vi "experiment control.vi"() -> ()   [LabVIEW 2012] (continued)
                          n671 = Enqueue Element At Opposite End(queue=w1523, element=w1521) -> ()  [unwired: 2 in, 3 out]
                        }
                        frame "Lasers" {
                          n672 = call "seek_tag.vi"("error in"=w1562, "Name"=w1563, "refnum"=w1561) -> ("error out"=w1559:errorcluster, "error"=w1552:string, "refnum"=w1560:refnum<file>)  [unwired: 6 in]
                          n673 = local read "Toptica"() -> (w1547:T19)
                          n674 = local read "Jessica"() -> (w1551:T17)
                          n675 = local read "Bertha"() -> (w1550:T22)
                          n676 = local read "Stella"() -> (w1548:T20)
                          n677 = local read "Cora"() -> (w1549:T21)
                          n678 = Concatenate Strings("Debug: Console >> " ("prompt (Open existing file)"), w1552) -> (w1543:string)
                          n679 = Bundle("Jessica"=w1551, "Bertha"=w1550, "Cora"=w1549, "Stella"=w1548, "Toptica"=w1547) -> (w1546:T88)  [unwired: 1 in]
                          n680 = call "ubinary.vi"("Cluster"=w1546) -> ("Header"=w1564:cluster{"Element Names":string[], u8[]})  [unwired: 9 in, 1 out]
                          n681 = Bundle("Header"=w1564, w1546) -> (w1557:T89)  [unwired: 1 in]
                          n682 = Read from Binary File(5:w1557, 8:w1559, 9:T45."native, host order" ("byte order (0:big-endian, network order)"), 11:w1560) -> (0:w1554:errorcluster, 2:w1555:T89, 3:w1556:refnum<file>)  [unwired: 2 in, 1 out]
                          n683 = case shown="No Error" w1554 {
                            tunnel: w1555 -> [w1571 _]
                            frame No Error {
                              n684 = Unbundle(w1571) -> (w1570:T88)  [unwired: 1 out]
                              n685 = Unbundle By Name(w1570) -> ("Jessica"=w1569:T17, "Bertha"=w1568:T22, "Cora"=w1567:T21, "Stella"=w1566:T20, "Toptica"=w1565:T19)
                              n686 = local write "Toptica"(w1565) -> ()
                              n687 = local write "Bertha"(w1568) -> ()
                              n688 = local write "Cora"(w1567) -> ()
                              n689 = local write "Stella"(w1566) -> ()
                              n690 = local write "Jessica"(w1569) -> ()
                            }
                            frame Error {
                            }
                          }
                          n691 = Enqueue Element At Opposite End(queue=w1544, element=w1543) -> ()  [unwired: 2 in, 3 out]
                        }
                        frame "AOM DDS" {
                          n692 = call "seek_tag.vi"("error in"=w1587, "Name"=w1588, "refnum"=w1586) -> ("error out"=w1584:errorcluster, "error"=w1577:string, "refnum"=w1585:refnum<file>)  [unwired: 6 in]
                          n693 = local read "DDS"() -> (w1576:T25)
                          n694 = Concatenate Strings("Debug: Console >> " ("prompt (Open existing file)"), w1577) -> (w1573:string)
                          n695 = Bundle("DDS"=w1576) -> (w1575:T66)  [unwired: 1 in]
                          n696 = call "ubinary.vi"("Cluster"=w1575) -> ("Header"=w1589:cluster{"Element Names":string[], u8[]})  [unwired: 9 in, 1 out]
                          n697 = Bundle("Header"=w1589, w1575) -> (w1582:T67)  [unwired: 1 in]
                          n698 = Read from Binary File(5:w1582, 8:w1584, 9:T45."native, host order" ("byte order (0:big-endian, network order)"), 11:w1585) -> (0:w1579:errorcluster, 2:w1580:T67, 3:w1581:refnum<file>)  [unwired: 2 in, 1 out]
                          n699 = case shown="No Error" w1579 {
                            tunnel: w1580 -> [w1592 _]
                            frame No Error {
                              n700 = Unbundle(w1592) -> (w1591:T66)  [unwired: 1 out]
                              n701 = Unbundle By Name(w1591) -> ("DDS"=w1590:T25)
                              n702 = local write "DDS"(w1590) -> ()
                            }
                            frame Error {
                            }
                          }
                          n703 = Enqueue Element At Opposite End(queue=w1572, element=w1573) -> ()  [unwired: 2 in, 3 out]
                        }
                        frame "Trap DDS" {
                          n704 = call "seek_tag.vi"("error in"=w1608, "Name"=w1609, "refnum"=w1607) -> ("error out"=w1605:errorcluster, "error"=w1598:string, "refnum"=w1606:refnum<file>)  [unwired: 6 in]
                          n705 = local read "Trap DDS"() -> (w1597:T26)
                          n706 = Concatenate Strings("Debug: Console >> " ("prompt (Open existing file)"), w1598) -> (w1594:string)
                          n707 = Bundle("Trap DDS"=w1597) -> (w1596:T68)  [unwired: 1 in]
                          n708 = call "ubinary.vi"("Cluster"=w1596) -> ("Header"=w1610:cluster{"Element Names":string[], u8[]})  [unwired: 9 in, 1 out]
                          n709 = Bundle("Header"=w1610, w1596) -> (w1603:T69)  [unwired: 1 in]
                          n710 = Read from Binary File(5:w1603, 8:w1605, 9:T45."native, host order" ("byte order (0:big-endian, network order)"), 11:w1606) -> (0:w1600:errorcluster, 2:w1601:T69, 3:w1602:refnum<file>)  [unwired: 2 in, 1 out]
                          n711 = case shown="No Error" w1600 {
                            tunnel: w1601 -> [w1613 _]
                            frame No Error {
                              n712 = Unbundle(w1613) -> (w1612:T68)  [unwired: 1 out]
                              n713 = Unbundle By Name(w1612) -> ("Trap DDS"=w1611:T26)
                              n714 = local write "Trap DDS"(w1611) -> ()
                            }
                            frame Error {
                            }
                          }
                          n715 = Enqueue Element At Opposite End(queue=w1593, element=w1594) -> ()  [unwired: 2 in, 3 out]
                        }
                        frame "Wavemaster" {
                          n716 = call "seek_tag.vi"("error in"=w1629, "Name"=w1630, "refnum"=w1628) -> ("error out"=w1626:errorcluster, "error"=w1619:string, "refnum"=w1627:refnum<file>)  [unwired: 6 in]
                          n717 = local read "Wavemaster"() -> (w1618:T23)
                          n718 = Concatenate Strings("Debug: Console >> " ("prompt (Open existing file)"), w1619) -> (w1614:string)
                          n719 = Bundle("Wavemaster"=w1618) -> (w1617:T76)  [unwired: 1 in]
                          n720 = call "ubinary.vi"("Cluster"=w1617) -> ("Header"=w1631:cluster{"Element Names":string[], u8[]})  [unwired: 9 in, 1 out]
                          n721 = Bundle("Header"=w1631, w1617) -> (w1624:T77)  [unwired: 1 in]
                          n722 = Read from Binary File(5:w1624, 8:w1626, 9:T45."native, host order" ("byte order (0:big-endian, network order)"), 11:w1627) -> (0:w1621:errorcluster, 2:w1622:T77, 3:w1623:refnum<file>)  [unwired: 2 in, 1 out]
                          n723 = case shown="No Error" w1621 {
                            tunnel: w1622 -> [w1634 _]
                            frame No Error {
                              n724 = Unbundle(w1634) -> (w1633:T76)  [unwired: 1 out]
                              n725 = Unbundle By Name(w1633) -> ("Wavemaster"=w1632:T23)
                              n726 = local write "Wavemaster"(w1632) -> ()
                            }
                            frame Error {
                            }
                          }
                          n727 = Enqueue Element At Opposite End(queue=w1615, element=w1614) -> ()  [unwired: 2 in, 3 out]
                        }
                        frame "Microwave" {
                          n728 = call "seek_tag.vi"("error in"=w1650, "Name"=w1651, "refnum"=w1649) -> ("error out"=w1647:errorcluster, "error"=w1640:string, "refnum"=w1648:refnum<file>)  [unwired: 6 in]
                          n729 = local read "HP8341B"() -> (w1639:T27)
                          n730 = Concatenate Strings("Debug: Console >> " ("prompt (Open existing file)"), w1640) -> (w1635:string)
                          n731 = Bundle("HP8341B"=w1639) -> (w1638:T78)  [unwired: 1 in]
                          n732 = call "ubinary.vi"("Cluster"=w1638) -> ("Header"=w1652:cluster{"Element Names":string[], u8[]})  [unwired: 9 in, 1 out]
                          n733 = Bundle("Header"=w1652, w1638) -> (w1645:T79)  [unwired: 1 in]
                          n734 = Read from Binary File(5:w1645, 8:w1647, 9:T45."native, host order" ("byte order (0:big-endian, network order)"), 11:w1648) -> (0:w1642:errorcluster, 2:w1643:T79, 3:w1644:refnum<file>)  [unwired: 2 in, 1 out]
                          n735 = case shown="No Error" w1642 {
                            tunnel: w1643 -> [w1655 _]
                            frame No Error {
                              n736 = Unbundle(w1655) -> (w1654:T78)  [unwired: 1 out]
                              n737 = Unbundle By Name(w1654) -> ("HP8341B"=w1653:T27)
                              n738 = local write "HP8341B"(w1653) -> ()
                            }
                            frame Error {
                            }
                          }
                          n739 = Enqueue Element At Opposite End(queue=w1636, element=w1635) -> ()  [unwired: 2 in, 3 out]
                        }
                        frame "Frequency" {
                          n740 = call "seek_tag.vi"("error in"=w1671, "Name"=w1672, "refnum"=w1670) -> ("error out"=w1668:errorcluster, "error"=w1661:string, "refnum"=w1669:refnum<file>)  [unwired: 6 in]
                          n741 = local read "Frequency Counter"() -> (w1660:T30)
                          n742 = Concatenate Strings("Debug: Console >> " ("prompt (Open existing file)"), w1661) -> (w1656:string)
                          n743 = Bundle("Frequency Counter"=w1660) -> (w1659:T82)  [unwired: 1 in]
                          n744 = call "ubinary.vi"("Cluster"=w1659) -> ("Header"=w1673:cluster{"Element Names":string[], u8[]})  [unwired: 9 in, 1 out]
                          n745 = Bundle("Header"=w1673, w1659) -> (w1666:T83)  [unwired: 1 in]
                          n746 = Read from Binary File(5:w1666, 8:w1668, 9:T45."native, host order" ("byte order (0:big-endian, network order)"), 11:w1669) -> (0:w1663:errorcluster, 2:w1664:T83, 3:w1665:refnum<file>)  [unwired: 2 in, 1 out]
                          n747 = case shown="No Error" w1663 {
                            tunnel: w1664 -> [w1676 _]
                            frame No Error {
                              n748 = Unbundle(w1676) -> (w1675:T82)  [unwired: 1 out]
                              n749 = Unbundle By Name(w1675) -> ("Frequency Counter"=w1674:T30)
                              n750 = local write "Frequency Counter"(w1674) -> ()
                            }
                            frame Error {
                            }
                          }
                          n751 = Enqueue Element At Opposite End(queue=w1657, element=w1656) -> ()  [unwired: 2 in, 3 out]
                        }
                        frame "Commands" {
                          n752 = local read "Measure Commands"() -> (w1684:string)
                          n753 = call "seek_tag.vi"("error in"=w1695, "Name"=w1696, "refnum"=w1694) -> ("error out"=w1692:errorcluster, "error"=w1685:string, "refnum"=w1693:refnum<file>)  [unwired: 6 in]
                          n754 = local read "Test Commands"() -> (w1683:string)
                          n755 = local read "Functions"() -> (w1682:cluster{"Name":string, "Body":string}[])
                          n756 = local read "Chops"() -> (w1679:cluster{"Chops":u16[]}[])
                          n757 = Concatenate Strings("Debug: Console >> " ("prompt (Open existing file)"), w1685) -> (w1677:string)
                          n758 = Bundle("Measure Commands"=w1684, "Test Commands"=w1683, "Functions"=w1682, "Chops"=w1679) -> (w1681:T70)  [unwired: 1 in]
                          n759 = call "ubinary.vi"("Cluster"=w1681) -> ("Header"=w1697:cluster{"Element Names":string[], u8[]})  [unwired: 9 in, 1 out]
                          n760 = Bundle("Header"=w1697, w1681) -> (w1690:T71)  [unwired: 1 in]
                          n761 = Read from Binary File(5:w1690, 8:w1692, 9:T45."native, host order" ("byte order (0:big-endian, network order)"), 11:w1693) -> (0:w1687:errorcluster, 2:w1688:T71, 3:w1689:refnum<file>)  [unwired: 2 in, 1 out]
                          n762 = case shown="No Error" w1687 {
                            tunnel: w1688 -> [w1703 _]
                            frame No Error {
                              n763 = Unbundle(w1703) -> (w1702:T70)  [unwired: 1 out]
                              n764 = Unbundle By Name(w1702) -> ("Measure Commands"=w1701:string, "Test Commands"=w1700:string, "Functions"=w1699:cluster{"Name":string, "Body":string}[], "Chops"=w1698:cluster{"Chops":u16[]}[])
                              n765 = local write "Measure Commands"(w1701) -> ()
                              n766 = local write "Test Commands"(w1700) -> ()
                              n767 = local write "Functions"(w1699) -> ()
                              n768 = local write "Chops"(w1698) -> ()
                            }
                            frame Error {
                            }
                          }
                          n769 = Enqueue Element At Opposite End(queue=w1678, element=w1677) -> ()  [unwired: 2 in, 3 out]
                        }
                        frame "Time" {
                          n770 = call "seek_tag.vi"("error in"=w1720, "Name"=w1721, "refnum"=w1719) -> ("error out"=w1717:errorcluster, "error"=w1710:string, "refnum"=w1718:refnum<file>)  [unwired: 6 in]
                          n771 = local read "Time"() -> (w1708:string)
                          n772 = local read "Date"() -> (w1709:string)
                          n773 = Concatenate Strings("Debug: Console >> " ("prompt (Open existing file)"), w1710) -> (w1704:string)
                          n774 = Bundle("Date"=w1709, "Time"=w1708) -> (w1707:cluster{"Date":string, "Time":string})  [unwired: 1 in]
                          n775 = call "ubinary.vi"("Cluster"=w1707) -> ("Header"=w1722:cluster{"Element Names":string[], u8[]})  [unwired: 9 in, 1 out]
                          n776 = Bundle("Header"=w1722, w1707) -> (w1715:T90)  [unwired: 1 in]
                          n777 = Read from Binary File(5:w1715, 8:w1717, 9:T45."native, host order" ("byte order (0:big-endian, network order)"), 11:w1718) -> (0:w1712:errorcluster, 2:w1713:T90, 3:w1714:refnum<file>)  [unwired: 2 in, 1 out]
                          n778 = case shown="No Error" w1712 {
                            tunnel: w1713 -> [w1726 _]
                            frame No Error {
                              n779 = Unbundle(w1726) -> (w1725:cluster{"Date":string, "Time":string})  [unwired: 1 out]
                              n780 = Unbundle By Name(w1725) -> ("Date"=w1724:string, "Time"=w1723:string)
                              n781 = local write "Time"(w1723) -> ()
                              n782 = local write "Date"(w1724) -> ()
                            }
                            frame Error {
                            }
                          }
                          n783 = Enqueue Element At Opposite End(queue=w1705, element=w1704) -> ()  [unwired: 2 in, 3 out]
                        }
                        frame "Switches" {
                          n784 = call "seek_tag.vi"("error in"=w1743, "Name"=w1744, "refnum"=w1742) -> ("error out"=w1740:errorcluster, "error"=w1733:string, "refnum"=w1741:refnum<file>)  [unwired: 6 in]
                          n785 = local read "Switch Settings"() -> (w1731:T9)
                          n786 = local read "Machine State"() -> (w1732:T1)
                          n787 = Concatenate Strings("Debug: Console >> " ("prompt (Open existing file)"), w1733) -> (w1727:string)
                          n788 = Bundle("Machine State"=w1732, "Switch Settings"=w1731) -> (w1730:T74)  [unwired: 1 in]
                          n789 = call "ubinary.vi"("Cluster"=w1730) -> ("Header"=w1745:cluster{"Element Names":string[], u8[]})  [unwired: 9 in, 1 out]
                          n790 = Bundle("Header"=w1745, w1730) -> (w1738:T75)  [unwired: 1 in]
                          n791 = Read from Binary File(5:w1738, 8:w1740, 9:T45."native, host order" ("byte order (0:big-endian, network order)"), 11:w1741) -> (0:w1735:errorcluster, 2:w1736:T75, 3:w1737:refnum<file>)  [unwired: 2 in, 1 out]
                          n792 = case shown="No Error" w1735 {
                            tunnel: w1736 -> [w1749 _]
                            frame No Error {
                              n793 = Unbundle(w1749) -> (w1748:T74)  [unwired: 1 out]
                              n794 = Unbundle By Name(w1748) -> ("Machine State"=w1747:T1, "Switch Settings"=w1746:T9)
                              n795 = local write "Switch Settings"(w1746) -> ()
                              n796 = local write "Machine State"(w1747) -> ()
                            }
                            frame Error {
                            }
                          }
                          n797 = Enqueue Element At Opposite End(queue=w1728, element=w1727) -> ()  [unwired: 2 in, 3 out]
                        }
                        frame "Data" {
                          n798 = call "seek_tag.vi"("error in"=w1770, "Name"=w1771, "refnum"=w1769) -> ("error out"=w1767:errorcluster, "error"=w1760:string, "refnum"=w1768:refnum<file>)  [unwired: 6 in]
                          n799 = local read "TDS5034B Oscilloscope"() -> (w1759:T24)
                          n800 = local read "TDS2014 Oscilloscope"() -> (w1758:T24)
                          n801 = Unbundle By Name(w1756) -> ("TDS5034B Data"=w1755:cluster{"Y":dbl[], "t0":dbl, "dt":dbl}[], "TDS2014 Data"=w1754:cluster{"Y":dbl[], "t0":dbl, "dt":dbl}[])
                          n802 = Concatenate Strings("Debug: Console >> " ("prompt (Open existing file)"), w1760) -> (w1750:string)
                          n803 = Bundle("TDS5034B Oscilloscope"=w1759, "TDS2014 Oscilloscope"=w1758, "TDS5034B Data"=w1755, "TDS2014 Data"=w1754) -> (w1757:T84)  [unwired: 1 in]
                          n804 = call "ubinary.vi"("Cluster"=w1757) -> ("Header"=w1772:cluster{"Element Names":string[], u8[]})  [unwired: 9 in, 1 out]
                          n805 = Bundle("Header"=w1772, w1757) -> (w1765:T85)  [unwired: 1 in]
                          n806 = Read from Binary File(5:w1765, 8:w1767, 9:T45."native, host order" ("byte order (0:big-endian, network order)"), 11:w1768) -> (0:w1762:errorcluster, 2:w1763:T85, 3:w1764:refnum<file>)  [unwired: 2 in, 1 out]
                          n807 = case shown="No Error" w1762 {
                            tunnel: w1763 -> [w1780 _]
                            tunnel: [w1776 w1781] -> w1753
                            tunnel: w1752 -> [w1773 w1781]
                            frame No Error {
                              n808 = Unbundle(w1780) -> (w1779:T84)  [unwired: 1 out]
                              n809 = Unbundle By Name(w1779) -> ("TDS5034B Oscilloscope"=w1778:T24, "TDS2014 Oscilloscope"=w1777:T24, "TDS5034B Data"=w1775:cluster{"Y":dbl[], "t0":dbl, "dt":dbl}[], "TDS2014 Data"=w1774:cluster{"Y":dbl[], "t0":dbl, "dt":dbl}[])
                              n810 = local write "TDS5034B Oscilloscope"(w1778) -> ()
                              n811 = local write "TDS2014 Oscilloscope"(w1777) -> ()
                              n812 = Bundle By Name(cluster=w1773, "TDS5034B Data"=w1775, "TDS2014 Data"=w1774) -> (w1776:T52)
                            }
                            frame Error {
                            }
                          }
                          n813 = Enqueue Element At Opposite End(queue=w1751, element=w1750) -> ()  [unwired: 2 in, 3 out]
                        }
                      }
                    }
                    n814 = Close File(refnum=w1450, error in=w1451) -> (error out=w1449:errorcluster)  [unwired: 1 out]
                  }
                }
              }
            }
          }
          frame "Begin Block" {
            # "Saves a uBinary file or loads a uBinary file."
            n815 = case shown="\"scan_switch\", Default" w1785 {
              selector: w1785 -> [w1790 _]
              tunnel: w1789 -> [w1791 w1801]
              tunnel: [w1791 w1802] -> w1788
              tunnel: [w1792 w1803] -> w1783
              tunnel: w1782 -> [_ w1800]
              frame "scan_switch", Default {
                n816 = Format Date/Time String(time format string (%c)="%Y") -> (date/time string=w1795:string)  [unwired: 2 in]
                n817 = Format Date/Time String(time format string (%c)="\\%y%m%d\\") -> (date/time string=w1793:string)  [unwired: 2 in]
                n818 = Concatenate Strings("X:\\" ("string"), w1795, w1793, w1790) -> (w1798:string)
                n819 = String To Path(string=w1798) -> (path=w1792:path)
              }
              frame "" {
                n820 = Format Date/Time String(time format string (%c)="%Y") -> (date/time string=w1813:string)  [unwired: 2 in]
                n821 = Format Date/Time String(time format string (%c)="\\%y%m%d\\") -> (date/time string=w1811:string)  [unwired: 2 in]
                n822 = Concatenate Strings("X:\\" ("string"), w1813, w1811) -> (w1817:string)
                n823 = String To Path(string=w1817) -> (path=w1815:path)
                n824 = call "File Dialog"("start path"=w1815, "error in"=w1801) -> ("selected path"=w1810:path, "cancelled"=w1799:bool, "error out"=w1802:errorcluster)  [unwired: 10 in, 1 out]
                n825 = Path To String(path=w1810) -> (string=w1804:string)
                n826 = case shown="True" w1799 {
                  tunnel: w1800 -> [_ w1818]
                  frame False {
                  }
                  frame True {
                    n827 = Flush Queue(queue=w1818) -> ()  [unwired: 1 in, 3 out]
                  }
                }
                n828 = xnode "Match Regular Expression"("input string"=w1804, "regular expression"="\\d$") -> ("before match"=w1805:string, "offset past match"=w1808:i32)  [unwired: 4 in, 3 out]
                n829 = Greater Or Equal To 0?(x=w1808) -> (x >= 0?=w1807:bool)
                n830 = Select(t=w1805, s=w1807, f=w1804) -> (s? t:f=w1806:string)
                n831 = String To Path(string=w1806) -> (path=w1803:path)
              }
            }
            n832 = Bundle By Name(cluster=w1787, "Block Index"=u32 1 ("Scan Index"), "Block Prefix"=w1783) -> (w1786:T52)
          }
          frame "Next Block" {
            # "Saves a uBinary file or loads a uBinary file."
            n833 = Unbundle By Name(w1933) -> ("Block Index"=w1932:u32)
            n834 = Increment(x=w1932) -> (x+1=w1931:u32)
            n835 = Bundle By Name(cluster=w1933, "Block Index"=w1931) -> (w1935:T52)
          }
          frame "Begin Scan" {
            # "Saves a uBinary file or loads a uBinary file."
            n836 = case shown="\"\", Default" w1944 {
              tunnel: w1943 -> [w1966 w2082]
              tunnel: [w1965 w2081] -> w1946
              tunnel: [w1957 FALSE ("cancelled")] -> w1937
              tunnel: [w1951 w2086] -> w1939
              tunnel: w1942 -> [w1948 w2079]
              tunnel: [w1948 w2080] -> w1938
              frame "", Default {
                n837 = Format Date/Time String(time format string (%c)="%Y") -> (date/time string=w1960:string)  [unwired: 2 in]
                n838 = Format Date/Time String(time format string (%c)="\\%y%m%d\\") -> (date/time string=w1958:string)  [unwired: 2 in]
                n839 = Concatenate Strings("X:\\" ("string"), w1960, w1958) -> (w1964:string)
                n840 = String To Path(string=w1964) -> (path=w1962:path)
                n841 = call "File Dialog6"("start path"=w1962, "error in"=w1966) -> ("selected path"=w1955:path, "cancelled"=w1957:bool, "error out"=w1965:errorcluster)  [unwired: 10 in, 1 out]
                n842 = Path To String(path=w1955) -> (string=w1950:string)
                n843 = xnode "Match Regular Expression"("input string"=w1950, "regular expression"="\\.ubin$") -> ("offset past match"=w1953:i32)  [unwired: 4 in, 4 out]
                n844 = Concatenate Strings(w1950, ".ubin" ("string")) -> (w1949:string)
                n845 = Greater Or Equal To 0?(x=w1953) -> (x >= 0?=w1952:bool)
                n846 = Select(t=w1950, s=w1952, f=w1949) -> (s? t:f=w1951:string)
              }
              frame "Block" {
                n847 = Unbundle By Name(w2079) -> ("Block Prefix"=w2087:path, "Block Index"=w2085:u32)
                n848 = while {
                  tunnel: w2087 -> [w2101]
                  tunnel: [w2097] -> w2083
                  shift-right: [w2092] -> w2081
                  shift-left: w2082 -> [w2096]
                  shift-right: [w2095] -> w2078
                  shift-left: w2085 -> [w2094]
                  stop <- w2089 continue-if-true
                  n849 = Path To String(path=w2101) -> (string=w2099:string)
                  n850 = Number To Decimal String(number=w2094) -> (decimal integer string=w2100:string)  [unwired: 1 in]
                  n851 = Concatenate Strings(w2099, w2100) -> (w2097:string)
                  n852 = String To Path(string=w2097) -> (path=w2098:path)
                  n853 = call <vilib>:"Check if File or Folder Exists.vi"("error in (no error)"=w2096, "path"=w2098) -> ("error out"=w2093:errorcluster, "file or folder exists?"=w2090:bool, "dup path"=w2091:path)  [unwired: 7 in]
                  n854 = case shown="True" w2090 {
                    selector: w2090 -> [w2102 _]
                    tunnel: w2093 -> [w2105 w2110]
                    tunnel: [w2104 w2109] -> w2092
                    tunnel: w2091 -> [w2103 w2111]
                    tunnel: [w2102 w2106] -> w2089
                    frame False {
                      n855 = Create Folder(path (use dialog)=w2103, error in=w2105) -> (error out=w2104:errorcluster)  [unwired: 1 in, 2 out]
                    }
                    frame True {
                      n856 = List Folder(path=w2111, error in=w2110) -> (filenames=w2108:string[], error out=w2109:errorcluster)  [unwired: 2 in, 2 out]
                      n857 = Array Size(array=w2108) -> (size(s)=w2107:i32)
                      n858 = Not Equal To 0?(x=w2107) -> (x != 0?=w2106:bool)
                    }
                  }
                  n859 = Increment(x=w2094) -> (x+1=w2095:u32)
                }
                n860 = Bundle By Name(cluster=w2079, "Block Index"=w2078) -> (w2080:T52)
                n861 = Concatenate Strings(w2083, "\\s.ubin" ("string")) -> (w2086:string)
              }
            }
            n862 = String To Path(string=w1939) -> (path=w1940:path)
            n863 = Bundle By Name(cluster=w1938, "Scan Index"=u32 0, "Scan Prefix"=w1940) -> (w1945:T52)
            n864 = case shown="True" w1937 {
              tunnel: w1936 -> [_ w1947]
              frame False {
              }
              frame True {
                n865 = Flush Queue(queue=w1947) -> ()  [unwired: 1 in, 3 out]
              }
            }
          }
          frame "Frames" {
            # "This command calls the custom functions specified in the programming tab"
            n866 = Index Array(array=w2114, index=0) -> (element=w2112:string)
            n867 = Index Array(array=w2114, index=1) -> (element=w2113:string)
            n868 = Decimal String To Number(string=w2113) -> (number=w2122:i32)  [unwired: 2 in, 1 out]
            n869 = Decimal String To Number(string=w2112) -> (number=w2126:i32)  [unwired: 2 in, 1 out]
            n870 = local read "TDS5034B Oscilloscope"() -> (w2121:T24)
            n871 = local read "Frames and Rep Rate"() -> (w2129:cluster{"Frames":i32, "Repetition Rate":dbl})
            n872 = In Range and Coerce(upper limit=250, x=w2126, lower limit=1) -> (coerced(x)=w2128:i32)  [unwired: 1 out]
            n873 = In Range and Coerce(upper limit=250, x=w2122, lower limit=1) -> (coerced(x)=w2120:i32)  [unwired: 1 out]
            n874 = Bundle By Name(cluster=w2129, "Frames"=w2128) -> (w2119:cluster{"Frames":i32, "Repetition Rate":dbl})
            n875 = Bundle By Name(cluster=w2121, "Frames"=w2120) -> (w2118:T24)
            n876 = local write "TDS5034B Oscilloscope"(w2118) -> ()
            n877 = local write "Frames and Rep Rate"(w2119) -> ()
          }
          frame "Scope: Frames" {
            # "This command calls the custom functions specified in the programming tab"
            n878 = Decimal String To Number(string=w2139) -> (number=w2136:i32)  [unwired: 2 in, 1 out]
            n879 = local read "TDS5034B Oscilloscope"() -> (w2135:T24)
            n880 = In Range and Coerce(upper limit=250, x=w2136, lower limit=1) -> (coerced(x)=w2134:i32)  [unwired: 1 out]
            n881 = Bundle By Name(cluster=w2135, "Frames"=w2134) -> (w2133:T24)
            n882 = local write "TDS5034B Oscilloscope"(w2133) -> ()
          }
          frame "DIO64: Frames" {
            # "This command calls the custom functions specified in the programming tab"
            n883 = Decimal String To Number(string=w2149) -> (number=w2144:i32)  [unwired: 2 in, 1 out]
            n884 = local read "Frames and Rep Rate"() -> (w2147:cluster{"Frames":i32, "Repetition Rate":dbl})
            n885 = In Range and Coerce(upper limit=250, x=w2144, lower limit=1) -> (coerced(x)=w2146:i32)  [unwired: 1 out]
            n886 = Bundle By Name(cluster=w2147, "Frames"=w2146) -> (w2148:cluster{"Frames":i32, "Repetition Rate":dbl})
            n887 = local write "Frames and Rep Rate"(w2148) -> ()
          }
          frame "MV500: Trigger" {
            # "This command calls the custom functions specified in the programming tab"
            n888 = Index Array(array=w2153) -> (element=w2152:string)  [unwired: 1 in]
            n889 = local read "Frames and Rep Rate"() -> (w2169:cluster{"Frames":i32, "Repetition Rate":dbl})
            n890 = case shown="\"True\"" w2152 {
              tunnel: w2156 -> [_ w2179]
              tunnel: ["" w2178] -> w2154
              frame "new", Default {
              }
              frame "True" {
                n891 = Unbundle By Name(w2179) -> ("Scan Prefix"=w2176:path, "Scan Index"=w2177:u32)
                n892 = Strip Path(path=w2176) -> (stripped path=w2175:path)  [unwired: 1 out]
                n893 = Number To Decimal String(number=w2177) -> (decimal integer string=w2174:string)  [unwired: 1 in]
                n894 = Path To String(path=w2175) -> (string=w2172:string)
                n895 = Concatenate Strings(w2172, "\\trap" ("string"), w2174) -> (w2178:string)
              }
            }
            n896 = TCP Open Connection(address="192.168.1.105", remote port or service name=u16 44444, error in (no error)=w2170) -> (connection ID=w2160:refnum<k5>, error out=w2168:errorcluster)  [unwired: 2 in]
            n897 = Unbundle By Name(w2169) -> ("Frames"=w2165:i32)
            n898 = Build Array(w2165) -> (w2164:i32[])
            n899 = Byte Array To String(unsigned byte array=w2164) -> (string=w2163:string)
            n900 = Concatenate Strings("MV" ("string"), w2163, w2154) -> (w2161:string)
            n901 = TCP Write(connection ID=w2160, data in=w2161, error in (no error)=w2168) -> (connection ID out=w2157:refnum<k5>, error out=w2158:errorcluster)  [unwired: 1 in, 1 out]
            n902 = Bundle By Name(cluster=w2156, "img mcp tcp"=w2157) -> (w2155:T52)
          }
          frame "IMG MCP: Clear" {
            # "This command calls the custom functions specified in the programming tab"
            n903 = local write "img_mcp:averages"(u32 0 ("img_mcp:averages")) -> ()
            n904 = local write "img mcp"(dbl[][] [] ("img mcp")) -> ()
          }
          frame "MV500: Read" {
            # "This command calls the custom functions specified in the programming tab"
            n905 = Unbundle By Name(w2202) -> ("img mcp tcp"=w2193:refnum<k5>)
            n906 = Multiply(x=480 ("bytes to read"), y=640 ("bytes to read")) -> (x*y=w2199:i32)
            n907 = TCP Read(connection ID=w2193, bytes to read=w2199, error in (no error)=w2192) -> (connection ID out=w2191:refnum<k5>, data out=w2198:string, error out=w2190:errorcluster)  [unwired: 2 in]
            n908 = Type Cast(type=u8[] [0], x=w2198) -> (*(type *) &x=w2196:u8[])
            n909 = Reshape Array(w2196, 480 ("dimension size"), 640 ("dimension size")) -> (w2188:u8[][])
            n910 = for {
              tunnel: w2188 -> [w2215] mode=indexing
              tunnel: [w2214] -> w2187 mode=indexing
              n911 = Reverse 1D Array(array=w2215) -> (reversed array=w2214:u8[])
            }
            n912 = Transpose 2D Array(2D array=w2187) -> (transposed array=w2186:u8[][])
            n913 = case shown="Default" "img_mcp:averages" {
              selector: "img_mcp:averages" -> [w2205 w2207]
              tunnel: w2186 -> [w2206 w2213]
              frame 0 {
                n914 = Increment(x=w2205) -> (x+1=w2204:u32)
                n915 = local write "img_mcp:averages"(w2204) -> ()
                n916 = local write "img mcp"(w2206) -> ()
              }
              frame Default {
                n917 = local read "img mcp"() -> (w2212:dbl[][])
                n918 = Multiply(x=w2212, y=w2207) -> (x*y=w2211:dbl[][])
                n919 = Increment(x=w2207) -> (x+1=w2209:u32)
                n920 = Add(x=w2211, y=w2213) -> (x+y=w2210:dbl[][])
                n921 = Divide(x=w2210, y=w2209) -> (x/y=→"img mcp":dbl[][])
                n922 = local write "img_mcp:averages"(w2209) -> ()
              }
            }
            n923 = TCP Close Connection(connection ID=w2191, error in (no error)=w2190) -> (error out=w2189:errorcluster)  [unwired: 1 in, 1 out]
          }
          frame "Move Down" {
            # "Saves a uBinary file or loads a uBinary file."
            n924 = Array Size(array=w2216) -> (size(s)=w2220:i32)
            n925 = Greater?(x=w2220, y=1) -> (0:w2217:bool)
            n926 = case shown="False" w2217 {
              tunnel: w2222 -> [w2227 w2273]
              tunnel: [w2226 w2272] -> w2221
              tunnel: w2218 -> [w2225 _]
              tunnel: w2216 -> [_ w2285]
              frame False {
                n927 = case shown="Default" w2225 {
                  selector: w2225 -> [_ w2235]
                  tunnel: w2227 -> [w2228 w2231]
                  tunnel: [w2228 w2238] -> w2226
                  frame "" {
                  }
                  frame Default {
                    n928 = local read "Working Directory"() -> (w2237:path)
                    n929 = Path To String(path=w2237) -> (string=w2234:string)
                    n930 = Concatenate Strings(w2234, "\\" ("string"), w2235) -> (w2233:string)
                    n931 = String To Path(string=w2233) -> (path=w2232:path)
                    n932 = call <vilib>:"Check if File or Folder Exists.vi"("error in (no error)"=w2231, "path"=w2232) -> ("error out"=w2230:errorcluster, "file or folder exists?"=w2229:bool)  [unwired: 7 in, 1 out]
                    n933 = case shown="True" w2229 {
                      tunnel: [w2241 w2246] -> w2238
                      tunnel: w2233 -> [w2240 w2243]
                      tunnel: w2230 -> [w2241 w2242]
                      frame True {
                        n934 = String To Path(string=w2240) -> (path=w2239:path)
                        n935 = local write "Working Directory"(w2239) -> ()
                      }
                      frame False {
                        n936 = while {
                          tunnel: w2243 -> [w2258]
                          tunnel: w2242 -> [w2255]
                          tunnel: [w2254] -> w2245
                          tunnel: [w2251] -> w2244
                          i -> [w2249]
                          stop <- w2250 stop-if-true
                          n937 = Increment(x=w2249) -> (x+1=w2248:i32)
                          n938 = Number To Decimal String(number=w2248) -> (decimal integer string=w2256:string)  [unwired: 1 in]
                          n939 = Concatenate Strings(w2258, w2256) -> (w2257:string)
                          n940 = String To Path(string=w2257) -> (path=w2252:path)
                          n941 = call <vilib>:"Check if File or Folder Exists.vi"("error in (no error)"=w2255, "path"=w2252) -> ("error out"=w2254:errorcluster, "file or folder exists?"=w2253:bool)  [unwired: 7 in, 1 out]
                          n942 = case shown="True" w2253 {
                            tunnel: w2252 -> [w2260 w2261]
                            tunnel: [w2260 w2261] -> w2251
                            tunnel: [TRUE w2262] -> w2250
                            frame False {
                            }
                            frame True {
                              n943 = List Folder(path=w2261) -> (filenames=w2266:string[], folder names=w2267:string[])  [unwired: 3 in, 2 out]
                              n944 = Array Size(array=w2266) -> (size(s)=w2268:i32)
                              n945 = Array Size(array=w2267) -> (size(s)=w2269:i32)
                              n946 = Equal To 0?(x=w2268) -> (x = 0?=w2265:bool)
                              n947 = Equal To 0?(x=w2269) -> (x = 0?=w2264:bool)
                              n948 = And(x=w2265, y=w2264) -> (x .and. y?=w2263:bool)
                              n949 = case shown="False" w2263 {
                                tunnel: [FALSE TRUE] -> w2262
                                frame False {
                                }
                                frame True {
                                }
                              }
                            }
                          }
                        }
                        n950 = Create Folder(path (use dialog)=w2244, error in=w2245) -> (created path=w2247:path, error out=w2246:errorcluster)  [unwired: 1 in, 1 out]
                        n951 = local write "Working Directory"(w2247) -> ()
                      }
                    }
                  }
                }
              }
              frame True {
                n952 = Index Array(array=w2285, index=0) -> (element=w2278:string)
                n953 = Index Array(array=w2285, index=1) -> (element=w2277:string)
                n954 = local read "Working Directory"() -> (w2282:path)
                n955 = Concatenate Strings(w2278, w2277) -> (w2276:string)
                n956 = Path To String(path=w2282) -> (string=w2280:string)
                n957 = Concatenate Strings(w2280, "\\" ("string"), w2276) -> (w2275:string)
                n958 = String To Path(string=w2275) -> (path=w2274:path)
                n959 = Create Folder(path (use dialog)=w2274, error in=w2273) -> (created path=w2279:path, error out=w2272:errorcluster)  [unwired: 1 in, 1 out]
                n960 = local write "Working Directory"(w2279) -> ()
              }
            }
          }
          frame "Move Up" {
            # "Saves a uBinary file or loads a uBinary file."
            n961 = local read "Working Directory"() -> (w2290:path)
            n962 = Path To String(path=w2290) -> (string=w2289:string)
            n963 = xnode "Match Regular Expression"("input string"=w2289, "regular expression"="\\\\\\w+$") -> ("before match"=w2287:string)  [unwired: 4 in, 4 out]
            n964 = String To Path(string=w2287) -> (path=w2286:path)
            n965 = local write "Working Directory"(w2286) -> ()
          }
          frame "Go Today" {
            # "Saves a uBinary file or loads a uBinary file."
            n966 = Format Date/Time String(time format string (%c)="%Y") -> (date/time string=w2415:string)  [unwired: 2 in]
            n967 = Format Date/Time String(time format string (%c)="\\%y%m%d\\") -> (date/time string=w2417:string)  [unwired: 2 in]
            n968 = Concatenate Strings("X:\\" ("string"), w2415, w2417) -> (w2412:string)
            n969 = String To Path(string=w2412) -> (path=w2411:path)
            n970 = call <vilib>:"Check if File or Folder Exists.vi"("error in (no error)"=w2406, "path"=w2411) -> ("error out"=w2407:errorcluster, "file or folder exists?"=w2410:bool, "dup path"=w2409:path)  [unwired: 7 in]
            n971 = case shown="False" w2410 {
              tunnel: w2409 -> [w2423 w2425]
              tunnel: [w2422 w2425] -> w2408
              tunnel: w2407 -> [w2421 w2424]
              tunnel: [w2420 w2424] -> w2405
              frame False {
                n972 = Create Folder(path (use dialog)=w2423, error in=w2421) -> (created path=w2422:path, error out=w2420:errorcluster)  [unwired: 1 in, 1 out]
              }
              frame True {
              }
            }
            n973 = local write "Working Directory"(w2408) -> ()
          }
          frame "Check Lasers" {
            # "Saves a uBinary file or loads a uBinary file."
            n974 = local read "Stella"() -> (w2437:T20)
            n975 = local read "Toptica"() -> (w2436:T19)
            n976 = local read "Jessica"() -> (w2435:T17)
            n977 = Unbundle By Name(w2437) -> ("locked"=w2430:bool)
            n978 = Unbundle By Name(w2436) -> ("locked"=w2429:bool)
            n979 = Unbundle By Name(w2435) -> ("locked"=w2427:bool)
            n980 = And(x=w2430, y=w2429) -> (x .and. y?=w2428:bool)
            n981 = And(x=w2428, y=w2427) -> (x .and. y?=w2426:bool)
            n982 = case shown="False" w2426 {
              tunnel: w2432 -> [w2440 w2441]
              tunnel: [w2439 w2441] -> w2431
              frame False {
                n983 = Enqueue Element At Opposite End(queue=w2440, element="Pause") -> (queue out=w2439:refnum<queue>)  [unwired: 2 in, 2 out]
              }
              frame True {
              }
            }
          }
          frame "Depletion Flip" {
            # "Saves a uBinary file or loads a uBinary file."
            n984 = String Length(string=w2443) -> (length=w2444:i32)
            n985 = Greater Than 0?(x=w2444) -> (x > 0?=w2442:bool)
            n986 = case shown="True" w2442 {
              tunnel: w2448 -> [w2450 w2459]
              tunnel: [w2450 w2458] -> w2447
              tunnel: w2446 -> [w2451 w2457]
              tunnel: [w2451 w2456] -> w2445
              tunnel: w2443 -> [_ w2452]
              frame False {
              }
              frame True {
                n987 = Concatenate Strings("USB DAQ: Digital Write >> 4," ("string"), w2452) -> (w2454:string)
                n988 = Build Array(w2454) -> (w2453:string[])
                n989 = call "queue_array_front.vi"("error in"=w2457, "array"=w2453, "queue in"=w2459) -> ("error out"=w2456:errorcluster, "queue out"=w2458:refnum<queue>)  [unwired: 7 in]
              }
            }
          }
          frame "Bertha Flip" {
            # "Saves a uBinary file or loads a uBinary file."
            n990 = String Length(string=w2461) -> (length=w2462:i32)
            n991 = Greater Than 0?(x=w2462) -> (x > 0?=w2460:bool)
            n992 = case shown="True" w2460 {
              tunnel: w2466 -> [w2468 w2479]
              tunnel: [w2468 w2478] -> w2465
              tunnel: w2464 -> [w2469 w2477]
              tunnel: [w2469 w2476] -> w2463
              tunnel: w2461 -> [_ w2472]
              frame False {
              }
              frame True {
                n993 = Decimal String To Number(string=w2472) -> (number=w2471:i32)  [unwired: 2 in, 1 out]
                n994 = Not Equal To 0?(x=w2471) -> (x != 0?=w2470:bool)
                n995 = local write "Bertha Flip"(w2470) -> ()
                n996 = Concatenate Strings("USB DAQ: Digital Write >> 3," ("string"), w2472) -> (w2474:string)
                n997 = Build Array(w2474) -> (w2473:string[])
                n998 = call "queue_array_front.vi"("error in"=w2477, "array"=w2473, "queue in"=w2479) -> ("error out"=w2476:errorcluster, "queue out"=w2478:refnum<queue>)  [unwired: 7 in]
              }
            }
          }
          frame "---------- Switches ----------" {
            # "Template Separator\n(You can make a copy of, or modify, this frame)"
          }
          frame "Switch: Scan Reset" {
            n999 = Bundle By Name(cluster=w2489, "Switch Scan Index"=0) -> (w2488:T52)
            n1000 = property on="State Hierarchy" class="LstBox (strict)"() -> ("Value"=w2486:i32[])  [unwired: 2 in, 2 out]
            n1001 = Array Size(array=w2486) -> (size(s)=w2485:i32)
            n1002 = Greater Than 0?(x=w2485) -> (x > 0?=w2484:bool)
            n1003 = case shown="True" w2484 {
              tunnel: w2483 -> [w2491 w2495]
              frame True {
                n1004 = Enqueue Element At Opposite End(queue=w2491, element="Switch: Scan Step") -> ()  [unwired: 2 in, 3 out]
              }
              frame False {
